vi "Tom_Bentham_FF.vi"() -> (5 "Plug in titles":string[](array[string]), 7 "Plug in values":string[](array[string]))   [LabVIEW 2010]
uses:
  Globals/Plug_in_data_global.vi
  Globals/Meas_global.vi
panel:
  out "min value":dbl format="%.2f"
  out "max value":dbl format="%.2f"
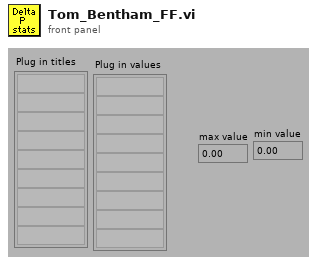
[diagram p1: front panel]
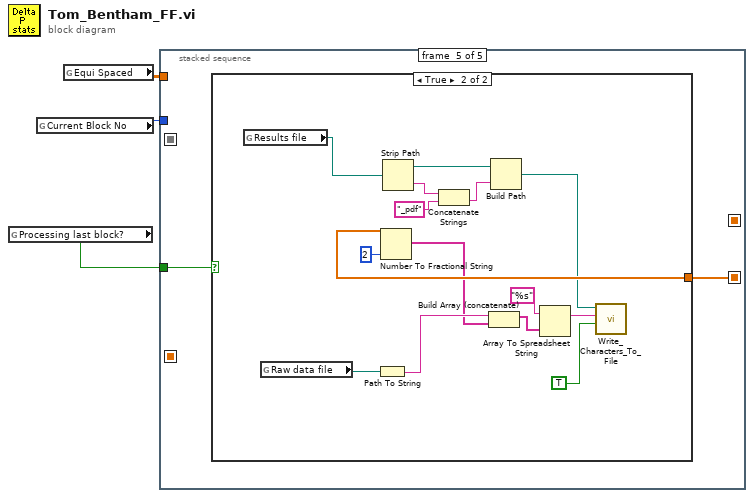
[diagram p0: block diagram]
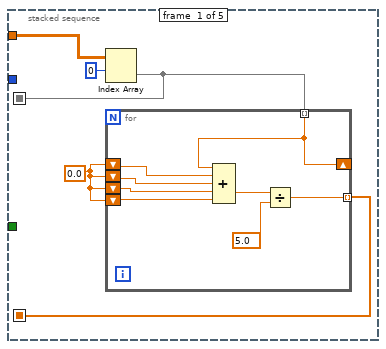
[diagram p2: hidden frame]
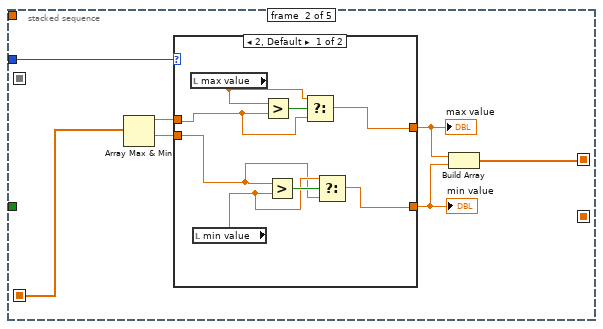
[diagram p3: hidden frame]
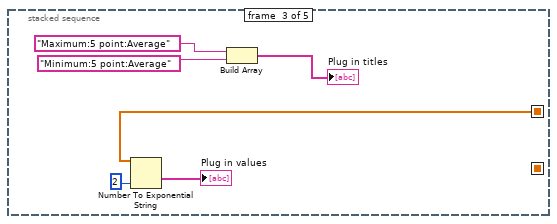
[diagram p5: hidden frame]
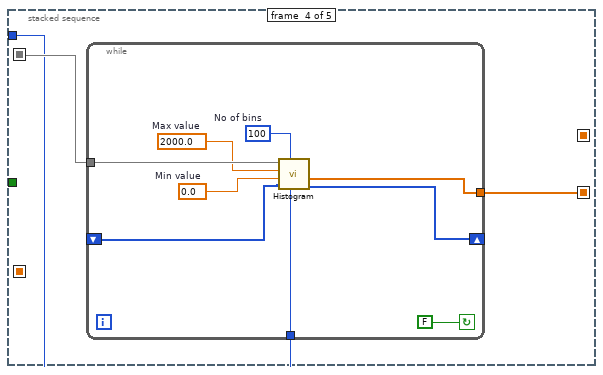
[diagram p6: hidden frame]
diagram:
  n1 = global read "Meas_global.vi" "Processing last block?"() -> (w1:bool)
  n2 = global read "Meas_global.vi" "Current Block No"() -> (w2:i32)
  n3 = global read "Plug_in_data_global.vi" "Equi Spaced"() -> (w3:dbl[][])
  n4 = stacked-sequence {
    seq-local: [w5 _ _ _ _] -> [_ w23 _ _ _]
    seq-local: [_ w18 _ _ _] -> [_ _ w35 _ _]
    seq-local: [w4 _ _ _ _] -> [_ _ _ w42 _]
    seq-local: [_ _ _ w41 _] -> [_ _ _ _ w52]
    tunnel: w3 -> [w7 _ _ _ _]
    tunnel: w2 -> [_ w17 _ w40 _]
    tunnel: w1 -> [_ _ _ _ w53]
    frame #0 {
      w6 = 0.0
      n5 = Index Array(array=w7, index (row)=0) -> (element=w4:dbl[])  [unwired: 1 in]
      n6 = for {
        shift-right: [w12] -> _
        shift-left: w6 -> [w16]
        shift-left: w6 -> [w15]
        shift-left: w6 -> [w14]
        shift-left: w6 -> [w13]
        tunnel: w4 -> [w12] mode=indexing
        tunnel: [w9] -> w5 mode=indexing
        n7 = Compound Arithmetic op=ADD(w12, w16, w15, w14, w13) -> (w11:dbl)
        n8 = Divide(x=w11, y=5.0) -> (x/y=w9:dbl)
      }
    }
    frame #1 {
      n9 = Array Max & Min(array=w23) -> (max value=w22:dbl, min value=w21:dbl)  [unwired: 2 out]
      n10 = case shown="2, Default" w17 {
        tunnel: [w28 w33] -> w20
        tunnel: w22 -> [w29 w33]
        tunnel: [w24 w32] -> w19
        tunnel: w21 -> [w25 w32]
        frame 2, Default {
          n11 = local read "max value"() -> (w30:dbl)
          n12 = local read "min value"() -> (w26:dbl)
          n13 = Greater?(x=w30, y=w29) -> (0:w31:bool)
          n14 = Greater?(x=w25, y=w26) -> (0:w27:bool)
          n15 = Select(t=w30, s=w31, f=w29) -> (s? t:f=w28:dbl)
          n16 = Select(t=w26, s=w27, f=w25) -> (s? t:f=w24:dbl)
        }
        frame 1 {
        }
      }
      "max value" <- w20
      "min value" <- w19
      n17 = Build Array(w20, w19) -> (w18:dbl[])
    }
    frame #2 {
      n18 = Number To Exponential String(number=w35, precision (6)=2) -> (E-format string=→"Plug in values":string[])  [unwired: 2 in]
      n19 = Build Array("Maximum:5 point:Average", "Minimum:5 point:Average") -> (→"Plug in titles":string[])
    }
    frame #3 {
      n20 = while {
        tunnel: w40 -> [w45]
        tunnel: [w46] -> w41
        shift-left: _ -> [w44]
        shift-right: [w49] -> _
        tunnel: w42 -> [w50]
        stop <- FALSE continue-if-true
        w47 = 2000.0  # Max value
        w48 = 0.0  # Min value
        w51 = 100  # No of bins
        n21 = call "Histogram.vi"("Current Block No"=w45, "No of bins"=w51, "Shift Hist"=w44, "Min value"=w48, "Max value"=w47, "X"=w50) -> ("Shift Hist"=w49:i32[], "Histogram of X"=w46:dbl[])  [unwired: 2 in, 1 out]
      }
    }
    frame #4 {
      n22 = case shown="True" w53 {
        tunnel: w52 -> [_ w68]
        frame False {
        }
        frame True {
          n23 = global read "Meas_global.vi" "Results file"() -> (w54:path)
          n24 = global read "Meas_global.vi" "Raw data file"() -> (w66:path)
          n25 = Path To String(path=w66) -> (string=w65:string)
          n26 = Number To Fractional String(number=w68, precision (6)=i16 2) -> (F-format string=w64:string[])  [unwired: 2 in]
          n27 = Strip Path(path=w54) -> (stripped path=w60:path, name=w59:string)
          n28 = Concatenate Strings(w59, "_pdf" ("Substring")) -> (w57:string)
          n29 = Build Array (concatenate)(w65, w64) -> (w63:string[])
          n30 = Build Path(base path=w60, name or relative path=w57) -> (appended path=w56:path)
          n31 = Array To Spreadsheet String(array=w63, 3:"%s" ("format string")) -> (spreadsheet string=w62:string)  [unwired: 1 in]
          n32 = call "Write_Characters_To_File.vi"("file path (dialog if empty)"=w56, "character string"=w62, "append to file? (new file:F)"=TRUE) -> ()  [unwired: 5 in, 1 out]
        }
      }
    }
  }
